vi "minorcheck.vi"(11 "Array in":bool[](array[boolean])) -> (3 "Array out":bool[](array[boolean]))   [LabVIEW 2019]
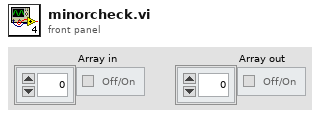
[diagram p1: front panel]
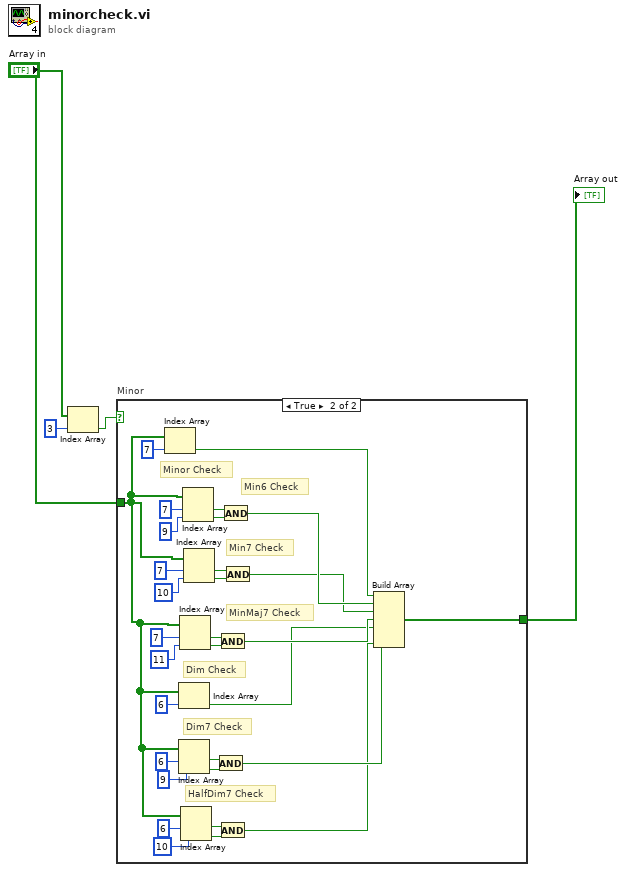
[diagram p0: block diagram]
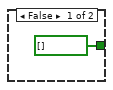
[diagram p2: hidden frame]
diagram:
  n1 = Index Array(array="Array in", index=3) -> (element=w2:bool)
  n2 = case "Minor" shown="True" w2 {
    tunnel: "Array in" -> [_ w14]
    tunnel: [bool[] [] w6] -> w3
    frame False {
    }
    frame True {
      # "HalfDim7 Check"
      # "Dim7 Check"
      # "Dim Check"
      # "MinMaj7 Check"
      # "Min6 Check"
      # "Min7 Check"
      # "Minor Check"
      n3 = Index Array(array=w14, index=7) -> (element=w13:bool)
      n4 = Index Array(array=w14, index=6) -> (element=w9:bool)
      n5 = Index Array(array=w14, index #1=6 ("index"), index #2=9 ("index")) -> (element #1=w19:bool, element #2=w21:bool)
      n6 = Index Array(array=w14, index #1=7 ("index"), index #2=11 ("index")) -> (element #1=w26:bool, element #2=w20:bool)
      n7 = Index Array(array=w14, index #1=6 ("index"), index #2=10 ("index")) -> (element #1=w18:bool, element #2=w17:bool)
      n8 = Index Array(array=w14, index #1=7 ("index"), index #2=9 ("index")) -> (element #1=w28:bool, element #2=w29:bool)
      n9 = Index Array(array=w14, index #1=7 ("index"), index #2=10 ("index")) -> (element #1=w33:bool, element #2=w32:bool)
      n10 = And(x=w19, y=w21) -> (x .and. y?=w8:bool)
      n11 = And(x=w26, y=w20) -> (x .and. y?=w10:bool)
      n12 = And(x=w18, y=w17) -> (x .and. y?=w7:bool)
      n13 = And(x=w28, y=w29) -> (x .and. y?=w12:bool)
      n14 = And(x=w33, y=w32) -> (x .and. y?=w11:bool)
      n15 = Build Array(w13, w12, w11, w10, w9, w8, w7) -> (w6:bool[])
    }
  }
  "Array out" <- w3
